vi "IND560 Convert String to Decimal.vi"(8 "Error In":errorcluster, 11 "read buffer":string) -> (0 "Error Out":errorcluster, 3 "Weigth":dbl)   [LabVIEW 2016]
uses:
  <vilib>/Utility/error.llb/whitespace.ctl
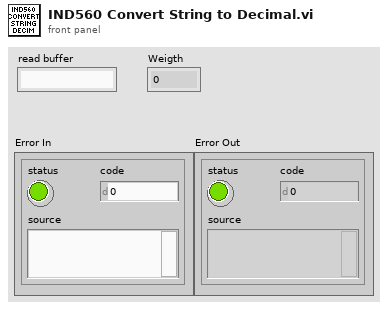
[diagram p1: front panel]
types:
  T1 = typedef "whitespace.ctl" = u16
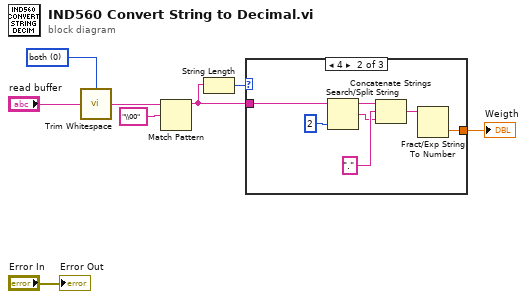
[diagram p0: block diagram]
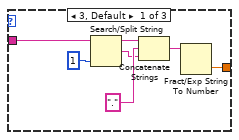
[diagram p2: hidden frame]
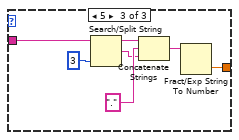
[diagram p3: hidden frame]
diagram:
  w7 = T1 0 items=["both", "start of string", "end of string"] ("location (both)")
  n1 = call <vilib>:"Trim Whitespace.vi"("string"="read buffer", "location (both)"=w7) -> ("trimmed string"=w3:string)
  n2 = Match Pattern(string=w3, regular expression="\\00" ("search string/char (-)")) -> (before substring=w1:string)  [unwired: 1 in, 3 out]
  n3 = String Length(string=w1) -> (length=w6:i32)
  n4 = case shown="4" w6 {
    tunnel: [w10 w16 w23] -> w5
    tunnel: w1 -> [w9 w17 w24]
    frame 3, Default {
      n5 = Search/Split String(string=w9, offset (0)=1) -> (substring before match=w14:string, match + rest of string=w12:string)  [unwired: 1 in, 1 out]
      n6 = Concatenate Strings(w14, "." ("string"), w12) -> (w11:string)
      n7 = Fract/Exp String To Number(string=w11) -> (number=w10:dbl)  [unwired: 3 in, 1 out]
    }
    frame 4 {
      n8 = Search/Split String(string=w17, offset (0)=2) -> (substring before match=w21:string, match + rest of string=w19:string)  [unwired: 1 in, 1 out]
      n9 = Concatenate Strings(w21, "." ("string"), w19) -> (w18:string)
      n10 = Fract/Exp String To Number(string=w18) -> (number=w16:dbl)  [unwired: 3 in, 1 out]
    }
    frame 5 {
      n11 = Search/Split String(string=w24, offset (0)=3) -> (substring before match=w28:string, match + rest of string=w26:string)  [unwired: 1 in, 1 out]
      n12 = Concatenate Strings(w28, "." ("string"), w26) -> (w25:string)
      n13 = Fract/Exp String To Number(string=w25) -> (number=w23:dbl)  [unwired: 3 in, 1 out]
    }
  }
  "Weigth" <- w5
  "Error Out" <- "Error In"
